vi "Test App Process Error Handler is Used if Configured.vi"(8 "error in (no error)":errorcluster, 11 "Rig Test In":refnum<class "Application Dev Test.lvclass">) -> (0 "error out":errorcluster, 3 "Rig Test Out":refnum<class "Application Dev Test.lvclass">)   [LabVIEW 2020, in "Application Dev Test.lvclass"]
uses:
  Application Dev Test.lvclass
  C:/Program Files (x86)/National Instruments/LabVIEW 2020/vi.lib/Astemes/LUnit/Test Case.lvclass
  source/Framework Test Suite/Mock Process/Mock Process.lvclass
  C:/Git/astemes-triarc-framework/source/Framework/Process/Process.lvclass
  source/Framework Test Suite/Mock Error Handler/Mock Error Handler.lvclass
  C:/Git/astemes-triarc-framework/source/Framework/Error Handler Interface/Error Handler Interface.lvclass
  source/Framework/Process/Process.lvclass/Process.ctl
  source/Framework/Application/Application.lvclass/Application.ctl
  <vilib>/Astemes/LUnit/Test Case.lvclass/Test Case.ctl
  <vilib>/Astemes/LUnit/LUnit Assertion Result.lvclass/LUnit Assertion Result.ctl
  <vilib>/Astemes/LUnit/LUnit Test Case Result.lvclass/LUnit Test Case Result.ctl
  <vilib>/Astemes/LUnit/LUnit Method Result.lvclass/LUnit Method Result.ctl
  4833bd43-5292-4b2f-bb91-aaf0710f4a92.vi
  source/Framework/Process/Protected/Messaging/Enqueue Message.vi
  source/Framework/Process/Public/Lifecycle/Get Lifecycle State.vi
  source/Framework/Application/Private/Add Process to Map.vi
  source/Framework/Application/Private/Start Idle Processes if Running.vi
  source/Framework/Application/Private/Throw Error If Process Already in App.vi
  source/Framework/Process/Protected/SubVIs/Set Context.vi
  source/Framework/Application/Private/Retrieve Process from App.vi
  source/Framework/Application/Private/Parse Process Name.vi
  source/Framework/Application/Private/Get Process from Map.vi
  <vilib>/Astemes/LUnit/Palette/Pass.vi
  <vilib>/Astemes/LUnit/Palette/Fail.vi
  <vilib>/Astemes/LUnit/Compare Variants.vi
  <vilib>/Astemes/LUnit/Describe Comparison.vi
  <vilib>/Astemes/LUnit/Set Assertion Type.vi
  source/Framework/Process/Private/SubVIs/Wait for finish.vi
  source/Framework/Process/Private/SubVIs/Set Lifecycle State.vi
  source/Framework/Process/Private/SubVIs/Handle Debug Data.vi
  <vilib>/Utility/error.llb/Clear Errors.vi
  source/Framework/Process/Public/Lifecycle/Leave Process Loop.vi
  source/Framework/Process/Protected/Messaging/Request Message.vi
  <vilib>/AdvancedString/Delimited String to 1D String Array.vi
  <vilib>/Astemes/LUnit/Add test result.vi
  <vilib>/Astemes/LUnit/LUnit Write Passed.vi
  <vilib>/Astemes/LUnit/LUnit Write Message.vi
  <vilib>/Astemes/LUnit/LUnit Write Description.vi
  <vilib>/Astemes/LUnit/Variant to string.vi
  <vilib>/Astemes/LUnit/LUnit Write Assertion Type.vi
  source/Framework/Logging/Log Debug.vi
  <vilib>/AdvancedString/1D String Array to Delimited String.vi
  <vilib>/Utility/High Resolution Relative Seconds.vi
  source/Framework/Process/Private/SubVIs/Enqueue Request Message.vi
  <vilib>/Astemes/LUnit/LUnit Record Assertion Result.vi
  <vilib>/Astemes/LUnit/LUnit Aggregate Assertion Results.vi
  <vilib>/Astemes/LUnit/Assertion Result/LUnit Read Status.vi
  <vilib>/Astemes/LUnit/LUnit Read Message.vi
  <vilib>/Astemes/LUnit/LUnit Read Description.vi
  <vilib>/Astemes/LUnit/Method Result/LUnit Merge Status.vi
  <vilib>/Astemes/LUnit/LUnit Concatenate result strings.vi
  source/Framework/Application/Application.lvclass
  <vilib>/Utility/error.llb/Error Cluster From Error Code.vi
  source/Framework/Process/Public/Read Name.vi
  source/Framework/Process/Private/SubVIs/Wait for Response Message.vi
  <vilib>/Utility/Data Type/Get Type Information.vi
  <vilib>/Utility/LVClass/Get LV Class Name.vi
  source/Framework/Process/Process.lvclass
  <vilib>/Astemes/LUnit/LUnit Assertion Result.lvclass
  <vilib>/Astemes/LUnit/Test Case.lvclass
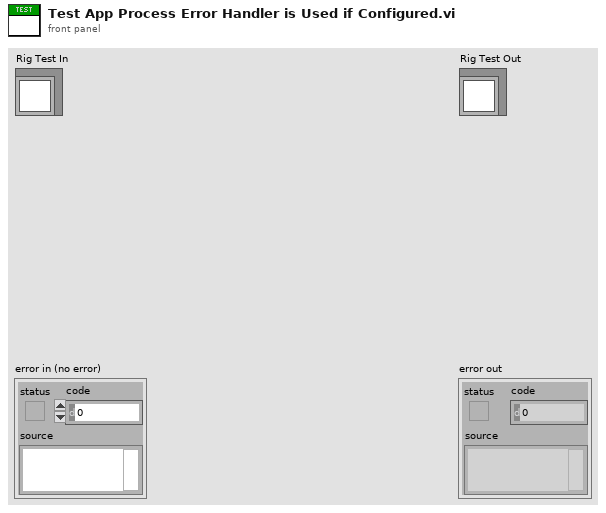
[diagram p1: front panel]
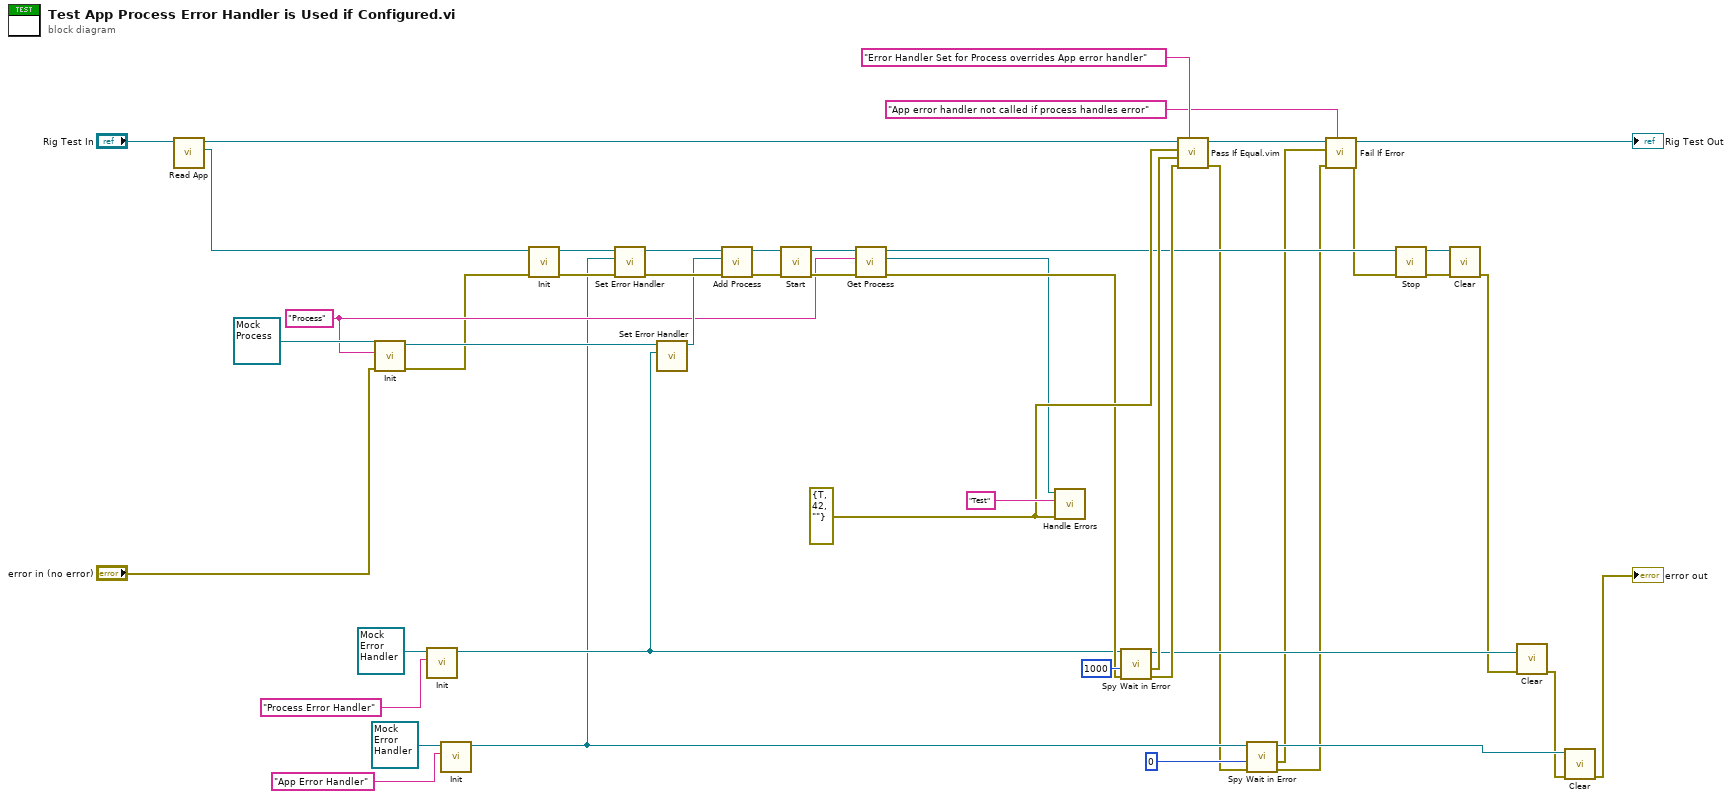
[diagram p0: block diagram]
diagram:
  w21 = "Process" ("Name")
  w40 = errorcluster {"status"=TRUE, "code"=42, "source"=""} ("error in (no error)")
  n1 = call "Read App.vi"("Application Test In"="Rig Test In") -> ("App out"=w31:refnum<class "Application.lvclass">, "Application Test Out"=w44:refnum<class "Application Dev Test.lvclass">)  [unwired: 8 in, 1 out]
  n2 = call-dynamic "Init.vi"("error in (no error)"="error in (no error)", "Name"=w21, "Mock Process In"=refnum<class "Mock Process.lvclass"> refnum ("Mock Process.lvclass")) -> ("error out"=w7:errorcluster, "Mock Process Out"=w19:refnum<class "Mock Process.lvclass">)  [unwired: 7 in]
  n3 = call-dynamic "Init.vi"("Name"="Process Error Handler", "Mock Error Handler In"=refnum<class "Mock Error Handler.lvclass"> refnum ("Mock Error Handler.lvclass")) -> ("Mock Error Handler Out"=w16:refnum<class "Mock Error Handler.lvclass">)  [unwired: 8 in, 1 out]
  n4 = call-dynamic "Init.vi"("Name"="App Error Handler", "Mock Error Handler In"=refnum<class "Mock Error Handler.lvclass"> refnum ("Mock Error Handler.lvclass")) -> ("Mock Error Handler Out"=w14:refnum<class "Mock Error Handler.lvclass">)  [unwired: 8 in, 1 out]
  n5 = call-dynamic "Init.vi"("error in (no error)"=w7, "Process In"=w31) -> ("error out"=w29:errorcluster, "Process Out"=w25:refnum<class "Application.lvclass">)  [unwired: 8 in]
  n6 = call "Set Error Handler.vi"("error in (no error)"=w29, "Error Handler"=w14, "Process In"=w25) -> ("error out"=w26:errorcluster, "Process Out"=w24:refnum<class "Application.lvclass">)  [unwired: 7 in]
  n7 = call "Set Error Handler.vi"("Error Handler"=w16, "Process In"=w19) -> ("Process Out"=w23:refnum<class "Mock Process.lvclass">)  [unwired: 8 in, 1 out]
  n8 = call "Add Process.vi"("error in (no error)"=w26, "Process"=w23, "Application In"=w24) -> ("error out"=w36:errorcluster, "Application Out"=w33:refnum<class "Application.lvclass">)  [unwired: 7 in]
  n9 = call "Start.vi"("error in (no error)"=w36, "Process In"=w33) -> ("error out"=w34:errorcluster, "Process Out"=w32:refnum<class "Application.lvclass">)  [unwired: 7 in, 1 out]
  n10 = call "Get Process.vi"("error in (no error)"=w34, "Process Name"=w21, "Application In"=w32) -> ("error out"=w27:errorcluster, "App Process"=w20:refnum<class "Process.lvclass">, "Application Out"=w28:refnum<class "Application.lvclass">)  [unwired: 6 in]
  n11 = call-dynamic "Handle Errors.vi"("error in (no error)"=w40, "Location"="Test", "Process In"=w20) -> ()  [unwired: 7 in, 2 out]
  n12 = call "Spy Wait in Error.vi"("error in (no error)"=w27, "timeout in ms (-1)"=1000, "Mock Error Handler In"=w16) -> ("error out"=w38:errorcluster, "Errors"=w39:errorcluster, "Mock Error Handler Out"=w13:refnum<class "Mock Error Handler.lvclass">)  [unwired: 4 in, 2 out]
  n13 = call "Pass If Equal.vim"("Description"="Error Handler Set for Process overrides App error handler", "error in (no error)"=w38, "Actual"=w39, "Expected"=w40, "LUnit Test Case In"=w44) -> ("error out"=w11:errorcluster, "LUnit Test Case Out"=w5:refnum<class "Application Dev Test.lvclass">)  [unwired: 5 in]
  n14 = call "Spy Wait in Error.vi"("error in (no error)"=w11, "timeout in ms (-1)"=0, "Mock Error Handler In"=w14) -> ("error out"=w3:errorcluster, "Errors"=w2:errorcluster, "Mock Error Handler Out"=w12:refnum<class "Mock Error Handler.lvclass">)  [unwired: 4 in, 2 out]
  n15 = call <vilib>:"Fail If Error.vi"("Description"="App error handler not called if process handles error", "error in (no error)"=w3, "Assert error"=w2, "LUnit Test Case In"=w5) -> ("error out"=w6:errorcluster, "LUnit Test Case Out"=→"Rig Test Out":refnum<class "Application Dev Test.lvclass">)  [unwired: 6 in]
  n16 = call "Stop.vi"("error in (no error)"=w6, "Process In"=w28) -> ("error out"=w30:errorcluster, "Process Out"=w35:refnum<class "Application.lvclass">)  [unwired: 7 in, 1 out]
  n17 = call-dynamic "Clear.vi"("error in (no error)"=w30, "Application In"=w35) -> ("error out"=w9:errorcluster)  [unwired: 9 in]
  n18 = call-dynamic "Clear.vi"("error in (no error)"=w9, "Mock Process In"=w13) -> ("error out"=w10:errorcluster)  [unwired: 9 in]
  n19 = call-dynamic "Clear.vi"("error in (no error)"=w10, "Mock Process In"=w12) -> ("error out"=→"error out":errorcluster)  [unwired: 9 in]
